vi "Initialize Entry.vi"(6 "chip select (1st)":enum16{"1st chip", "2nd chip"}(ring), 8 "error in (no error)":errorcluster, 11 "device index":i8) -> (0 "error out":errorcluster, 3 "LCD out":u32)   [LabVIEW 2015, in "HD44780 FPGA.lvlib"]
uses:
  <vilib>/EmbeddedDisplay/Hitachi HD44780/FPGA/HD44780 FPGA.lvlib
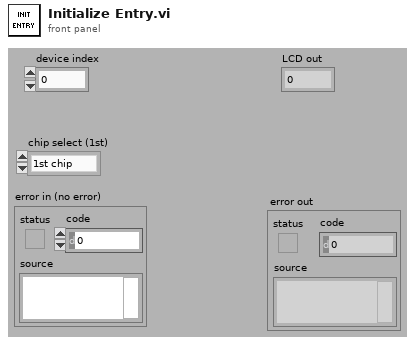
[diagram p1: front panel]
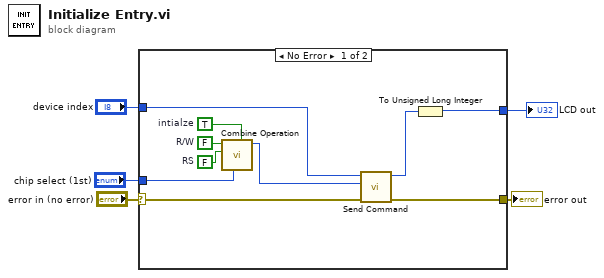
[diagram p0: block diagram]
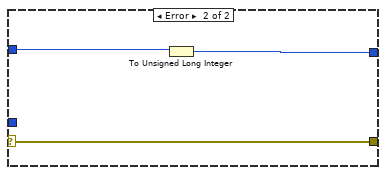
[diagram p2: hidden frame]
diagram:
  n1 = case shown="No Error" "error in (no error)" {
    selector: "error in (no error)" -> [w11 w18]
    tunnel: [w15 w18] -> w5
    tunnel: "device index" -> [w13 w17]
    tunnel: "chip select (1st)" -> [w12 _]
    tunnel: [w6 w16] -> w1
    frame No Error {
      w8 = TRUE  # intialze
      w9 = FALSE  # R/W
      w10 = FALSE  # RS
      n2 = call <vilib>:"Combine Operation.vi"("initialize entry (F)"=w8, "chip select  (1st chip)"=w12, "RS"=w10, "R/W"=w9) -> ("output"=w14:u32)  [unwired: 7 in]
      n3 = call <vilib>:"Send Command.vi"("error in (no error)"=w11, "operation"=w14, "device index"=w13) -> ("error out"=w15:errorcluster, "device index out"=w7:i8)  [unwired: 6 in, 1 out]
      n4 = To Unsigned Long Integer(number=w7) -> (unsigned 32bit integer=w6:u32)
    }
    frame Error {
      n5 = To Unsigned Long Integer(number=w17) -> (unsigned 32bit integer=w16:u32)
    }
  }
  "error out" <- w5
  "LCD out" <- w1
